vi "TTA_MATLAB_RX_Perform1RFIC1RxOutputPowerTest.vi"(0 "Channel":string(combo), 1 "MXG VISA Resource In":refnum<visa-resource-name>, 2 "EXA VISA Resource":refnum<visa-resource-name>, 5 "Rx":string(combo), 11 "error in":errorcluster) -> (4 "Output Power\nResults":T1, 12 "MXG VISA Resource Out":refnum<visa-resource-name>, 13 "EXA VISA Resource Out":refnum<visa-resource-name>, 15 "error out":errorcluster)   [LabVIEW 2016]
uses:
  TTA_Globals/TTA_Global_Complete_Settings.vi
panel:
  out "End Temp":dbl
  out "Start Temp":dbl
  out "In Range?":bool[](array[boolean])
  out "Amp Max\nSpec (dBm)":dbl
  out "Amp Min\nSpec (dBm)":dbl
  out "Frequency":dbl[](array[numeric])
  out "Amplitude":dbl[](array[numeric])
  out "IF Index":i32
  in  "PALLinearization Values":T2
  out "Rx#":i32
  out "CH#":i32
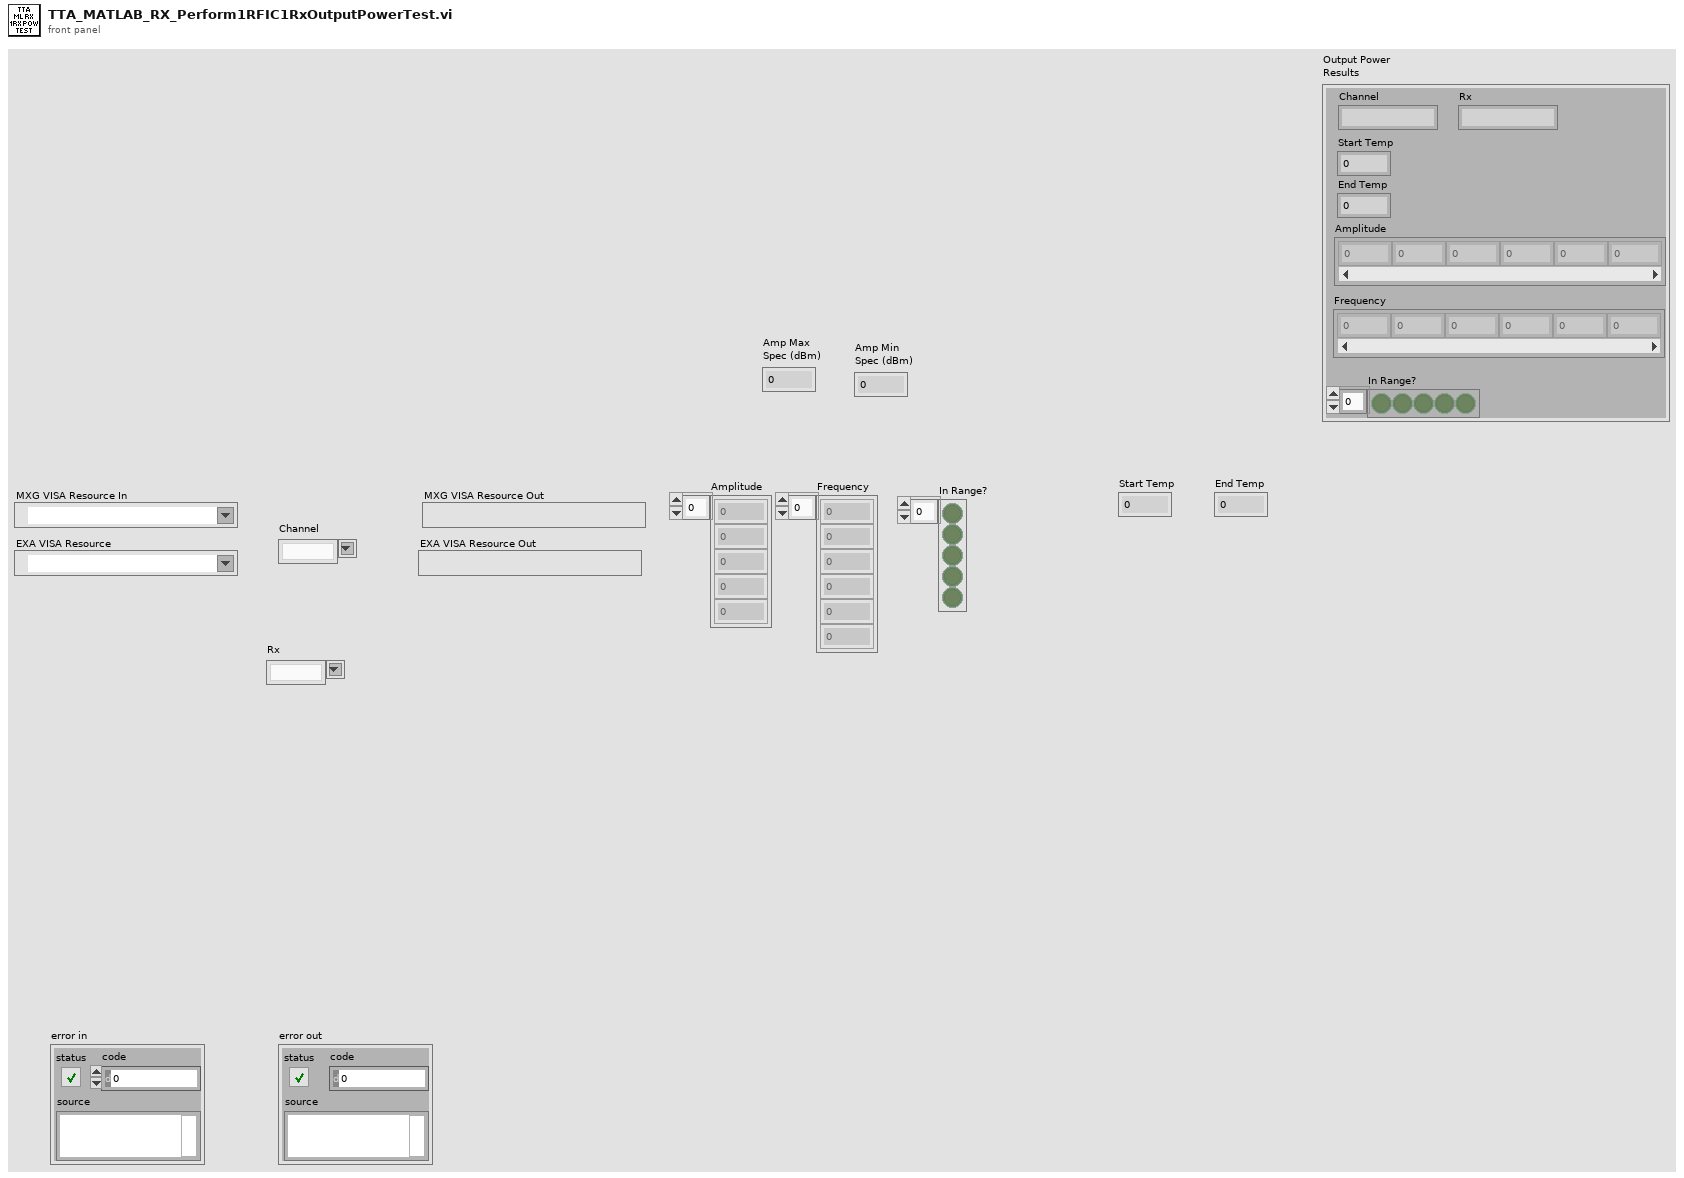
[diagram p1: front panel]
types:
  T1 = cluster{"Channel":string, "Rx":string, "Start Temp":dbl, "End Temp":dbl, "Amplitude":dbl[], "Frequency":dbl[], "In Range?":bool[]}
  T2 = cluster{"Tx IF Offsets":dbl[], "ACPR Filename":string, "Sampling Rate":dbl, "TxIF_Freq":dbl, "Power (dBm)":dbl, "IF Frequency Sweep (MHz)":dbl[], "BDSFreq":dbl, "Amplitude Range\nMax(dBm)":dbl, "Amplitude Range\nMin(dBm)":dbl, "CAL Amplitude\nIncrement(dB)":dbl, "CAL Amplitude\nDecrement (dB)":dbl, "Amplitude Least\nCriteria (dBm)":dbl}
  T3 = typedef "TTA_Control_Complete_Settings_Cluster.ctl" = cluster{"Brief Cluster":cluster{"STM Firmware File":string, "STM Firmware Address":string, "Required SW Version":string, "Template Used":string}, "Instrument Setting Cluster":cluster{"BDSFreq":dbl, "BDS Amp":dbl, "TxRFCal_Freq":dbl, "TxRFCal_Amp":dbl, "RxRFCal_Freq":dbl, "RxRFCal_Freq":dbl, "TxIF_Freq":dbl, "TxIF_Amp":dbl, "Tx_Output_Power_Signal_Freq":dbl, "Tx_ACPR_Signal_Freq":dbl, "Rx_RF_Freq":dbl, "Rx_RF_Amp":dbl, "Rx_Output_Power_Signal_Freq":dbl, "Rx_Output_Power_Sense_Freq":dbl}, "PAL Calibration\nInputs Cluster":cluster{"Amplitude Range\nMax(dBm)":dbl, "Amplitude Range\nMin(dBm)":dbl, "Amplitude Least\nCriteria (dBm)":dbl, "Frequency 1":dbl, "Frequency 2":dbl, "Frequency 3":dbl, "CAL Amplitude\nDecrement (dB)":dbl, "CAL Amplitude\nIncrement(dB)":dbl, "DownloadFile":string}, "TxOffset Cal Cluster":cluster{"Tx1 Offset (dB)":dbl, "Tx2 Offset (dB)":dbl, "Tx3 Offset (dB)":dbl, "Tx4 Offset (dB)":dbl, "Total RF Tx Loss (dB)":dbl}, "RxOffset Cal Cluster":cluster{"Rx1 Offset (dB)":dbl, "Rx2 Offset (dB)":dbl, "Rx3 Offset (dB)":dbl, "Rx4 Offset (dB)":dbl, "Total RF Rx Loss (dB)":dbl}, "TX Output Power Settings Cluster":cluster{"Frequency Sweep (MHz)":dbl[], "Sig Gen \nPower (dBm)":dbl, "Span (kHz)":dbl, "RBW (Hz)":dbl, "Ref Level (dBm)":dbl, "Low Power \nLimit":dbl, "High Power \nLimit":dbl, "DigAtt Max":dbl, "DigAtt Min":dbl}, "Tx ACPR Settings Cluster":cluster{"ACPR Filename":string, "Sampling Rate":dbl, "Power (dBm)":dbl, "IF Frequency Sweep (MHz)":dbl[], "State Name":string, "Mechanical\nAttenuation":dbl, "RefLevel Offset":dbl, "Amplitude Range\nMax (dBm)":dbl, "Amplitude Range\nMin (dBm)":dbl, "Cal Amp \nIncrement (dB)":dbl, "Cal Amp\nDecrement (dB)":dbl}, "Power Cal Cluster":cluster{"Power List (dBm)":dbl[], "Frequency (MHz)":dbl[], "Cal Decrement (dB)":dbl, "Cal Increment (dB)":dbl}, "Rx Received Power Settings Cluster":cluster{"Frequency Sweep (MHz)":dbl[], "Power (dBm)":dbl, "Span (kHz)":dbl, "RBW (Hz)":dbl, "Ref Level":dbl, "Low Power \nLimit (dBm)":dbl, "High Power\nLimit (dBm)":dbl}, "Tx Output Power Criteria Cluster":cluster{"CH1-TX1 \nMin":dbl, "CH1-TX1\nMax":dbl, "CH1-TXx3\nMin ":dbl, "CH1-TXx3\nMax":dbl, "CH2-TX1\nMin":dbl, "CH2-TX1\nMax":dbl, "CH2-TXx3\nMin":dbl, "CH2-TXx3\nMax":dbl}, "Tx ACPR Criteria Cluster":cluster{"Min Inband":dbl, "Max Close Outband":dbl, "Max Far Outband":dbl}, "Rx Output Power Criteria Cluster":cluster{"CH1-RX1 \nMin":dbl, "CH1-RX1 \nMax":dbl, "CH1-RXx3 \nMin":dbl, "CH1-RXx3\nMax":dbl, "CH2-RX1\nMin":dbl, "CH2-RX1\nMax":dbl, "CH2-RXx3\nMin":dbl, "CH2-RXx3\nMax":dbl}}
  T4 = cluster{"BDSFreq":dbl, "BDS Amp":dbl, "TxRFCal_Freq":dbl, "TxRFCal_Amp":dbl, "RxRFCal_Freq":dbl, "RxRFCal_Freq":dbl, "TxIF_Freq":dbl, "TxIF_Amp":dbl, "Tx_Output_Power_Signal_Freq":dbl, "Tx_ACPR_Signal_Freq":dbl, "Rx_RF_Freq":dbl, "Rx_RF_Amp":dbl, "Rx_Output_Power_Signal_Freq":dbl, "Rx_Output_Power_Sense_Freq":dbl}
  T5 = cluster{"Rx1 Offset (dB)":dbl, "Rx2 Offset (dB)":dbl, "Rx3 Offset (dB)":dbl, "Rx4 Offset (dB)":dbl, "Total RF Rx Loss (dB)":dbl}
  T6 = cluster{"Frequency Sweep (MHz)":dbl[], "Power (dBm)":dbl, "Span (kHz)":dbl, "RBW (Hz)":dbl, "Ref Level":dbl, "Low Power \nLimit (dBm)":dbl, "High Power\nLimit (dBm)":dbl}
  T7 = cluster{"CH1-RX1 \nMin":dbl, "CH1-RX1 \nMax":dbl, "CH1-RXx3 \nMin":dbl, "CH1-RXx3\nMax":dbl, "CH2-RX1\nMin":dbl, "CH2-RX1\nMax":dbl, "CH2-RXx3\nMin":dbl, "CH2-RXx3\nMax":dbl}
  T8 = enum16{"TX1", "TX2", "TX3", "TX4", "TXx3", "TXx4", "RX1", "RX2", "RX3", "RX4", "RXx3", "RXx4", "RFCal"}
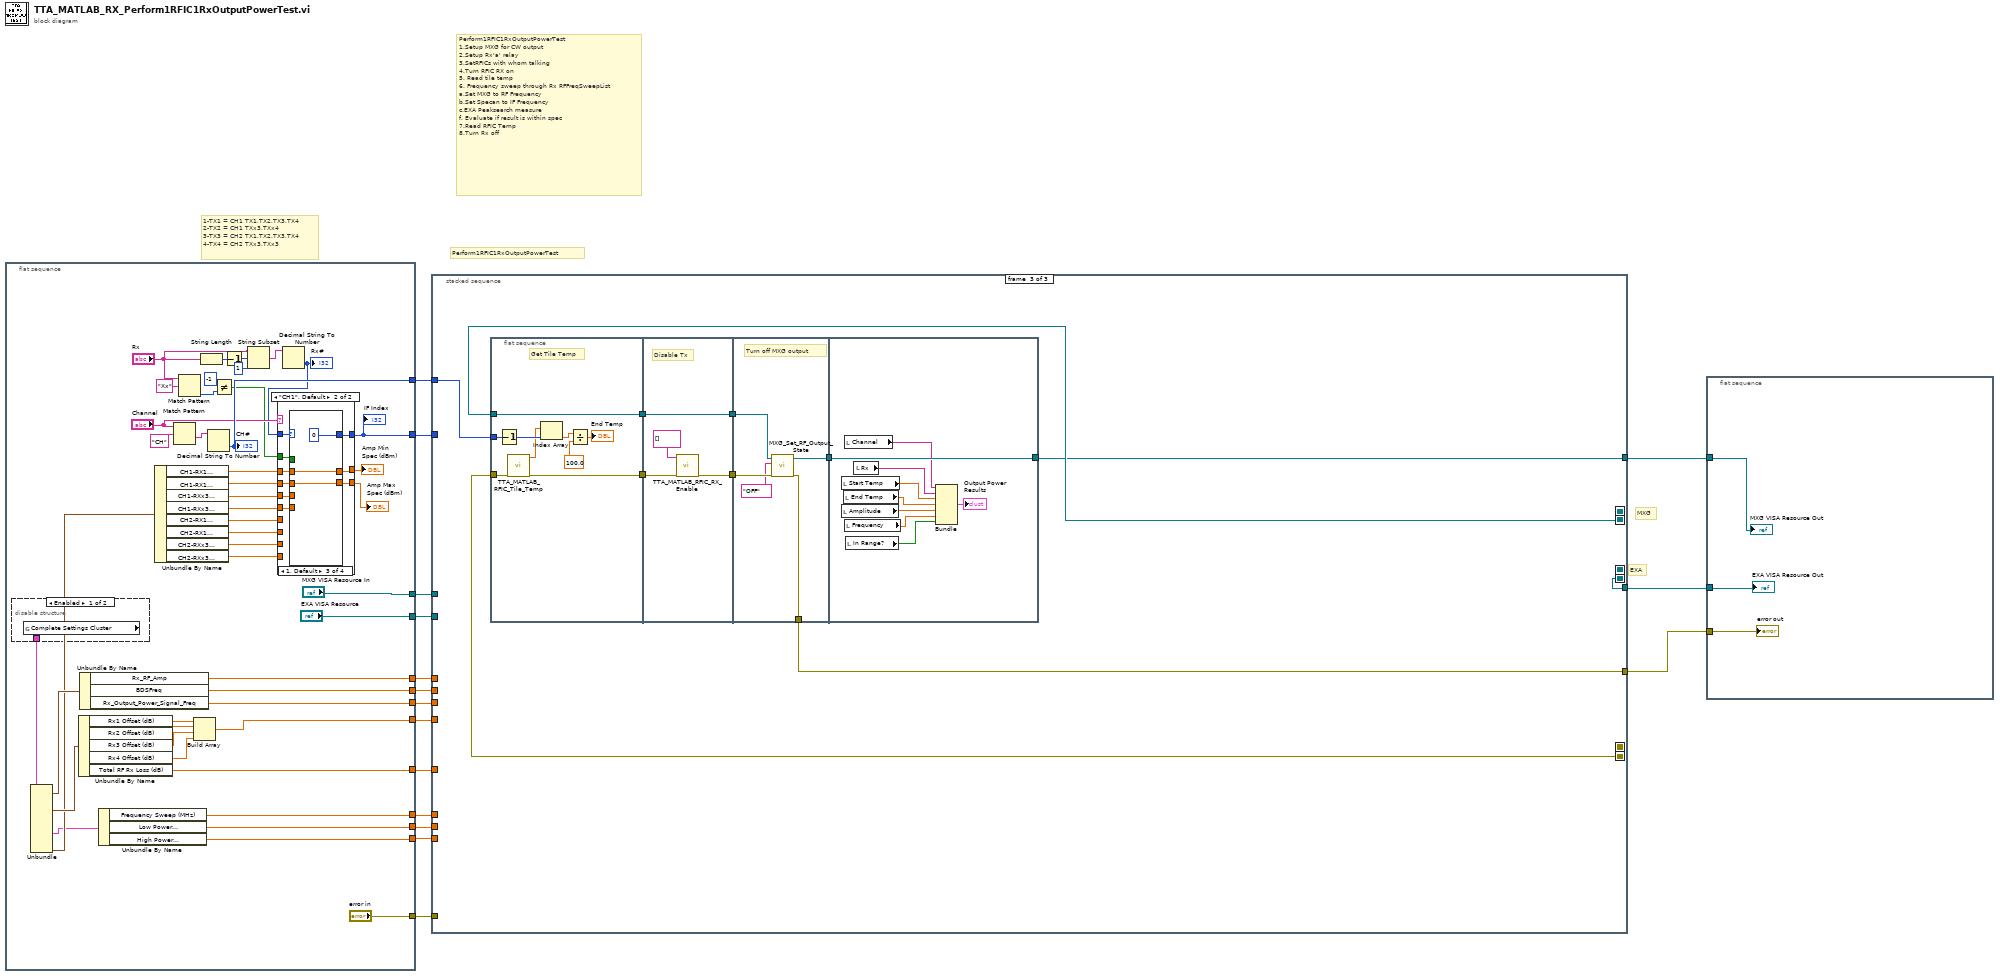
[diagram p0: block diagram]
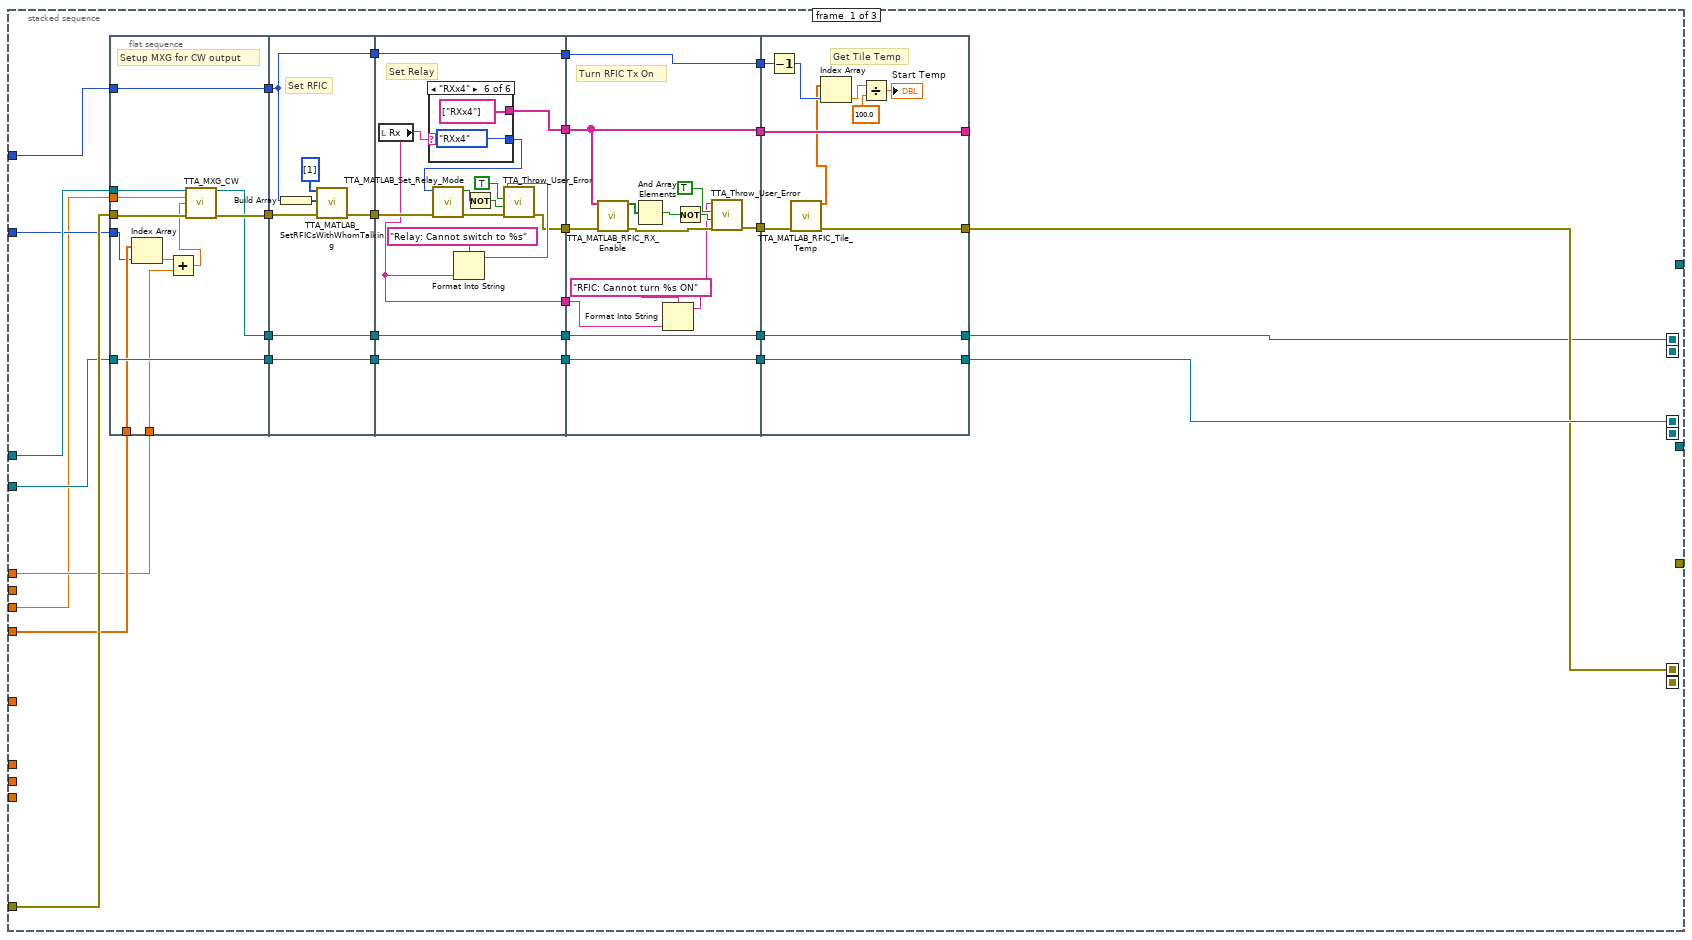
[diagram p2: hidden frame]
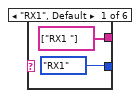
[diagram p3: hidden frame]
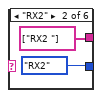
[diagram p4: hidden frame]
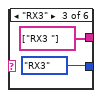
[diagram p5: hidden frame]
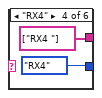
[diagram p6: hidden frame]
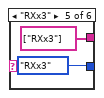
[diagram p7: hidden frame]
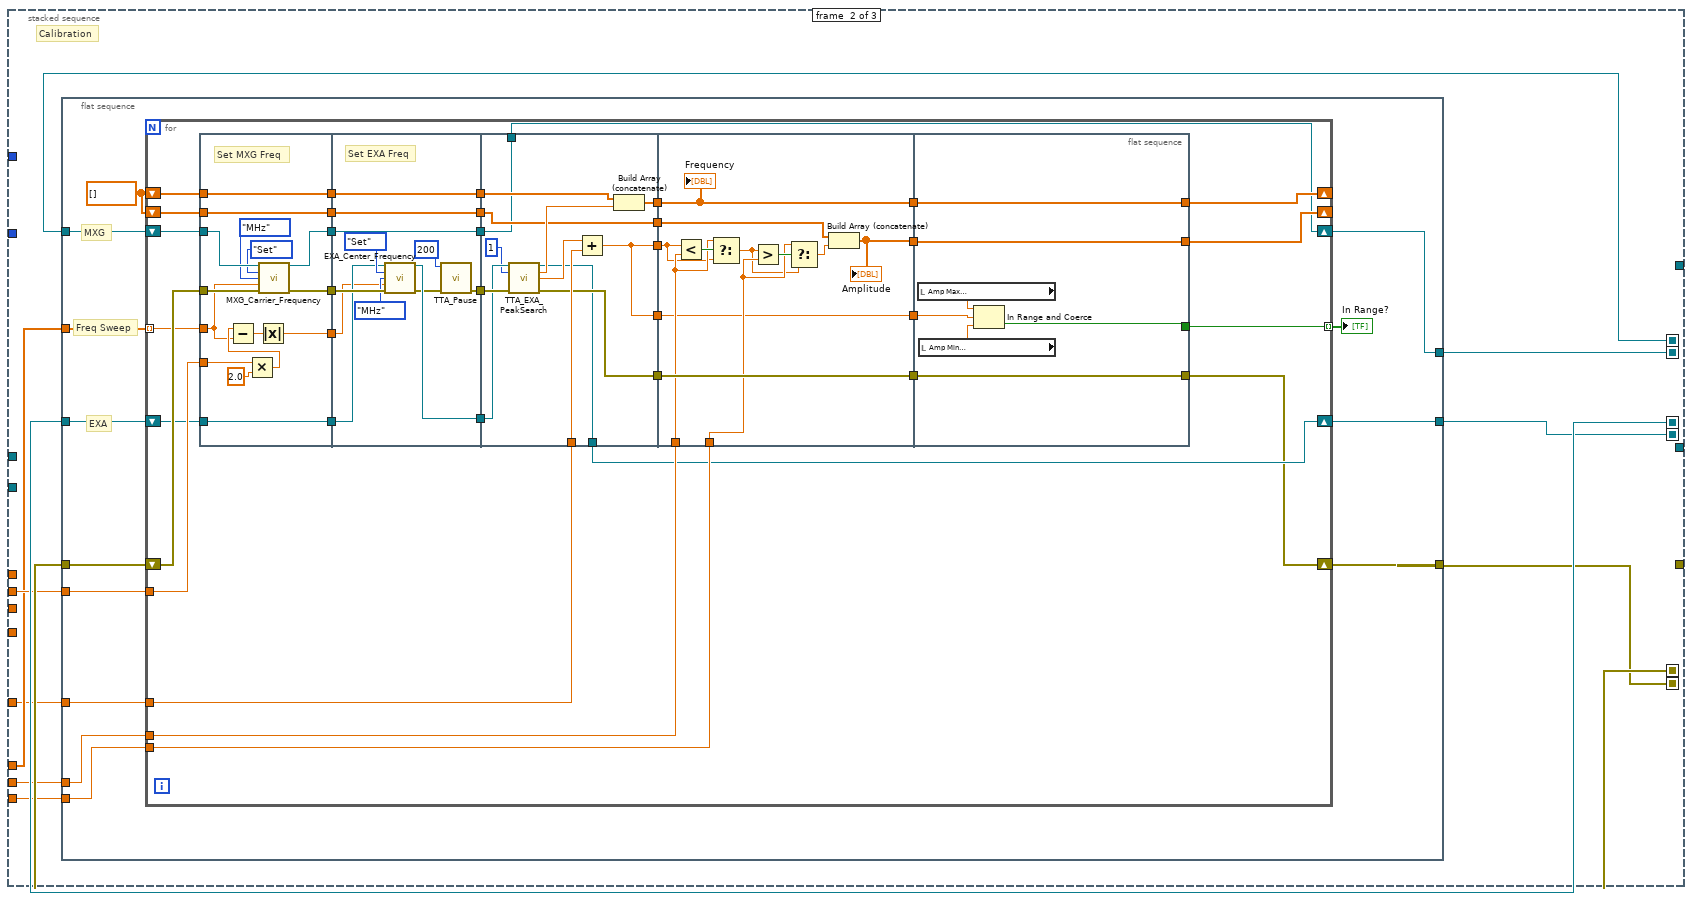
[diagram p8: hidden frame]
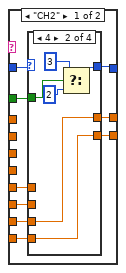
[diagram p9: hidden frame]
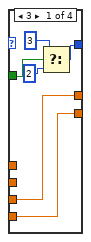
[diagram p10: hidden frame]
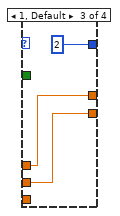
[diagram p11: hidden frame]
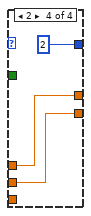
[diagram p12: hidden frame]
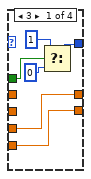
[diagram p13: hidden frame]
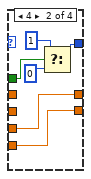
[diagram p14: hidden frame]
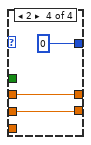
[diagram p15: hidden frame]
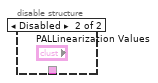
[diagram p16: hidden frame]
diagram:
  # "Perform1RFIC1RxOutputPowerTest\n1.Setup MXG for CW output\n2.Setup Rx'a' relay\n3.SetRFICs with whom talking\n4.Turn RFIC RX on\n5. Read tile temp\n6. Frequency sweep through Rx RFFreqSweepList\na.Set MXG to RF Frequency\nb.Set Specan to IF Frequency\nc.EXA Peaksearch measure\nf. Evaluate if result is within spec\n7.Read RFIC Temp\n8.Turn Rx off"
  # "Perform1RFIC1RxOutputPowerTest"
  # "1-TX1 = CH1 TX1,TX2,TX3,TX4\n2-TX2 = CH1 TXx3,TXx4\n3-TX3 = CH2 TX1,TX2,TX3,TX4\n4-TX4 = CH2 TXx3,TXx3"
  # "EXA"
  # "MXG"
  n1 = flat-sequence {
    tunnel: ["error in"] -> w16
    tunnel: ["MXG VISA Resource In"] -> w14
    tunnel: ["EXA VISA Resource"] -> w13
    tunnel: [w56] -> w15
    tunnel: [w43] -> w10
    tunnel: [w44] -> w9
    tunnel: [w49] -> w8
    tunnel: [w35] -> w7
    tunnel: [w34] -> w6
    tunnel: [w33] -> w5
    tunnel: [w32] -> w4
    tunnel: [w31] -> w3
    tunnel: [w30] -> w2
    frame #0 {
      n2 = disable-structure shown="Enabled" {
        disable-tunnel: [w116 _] -> w51
        frame Enabled {
          n3 = global read "TTA_Global_Complete_Settings.vi" "Complete Settings Cluster"() -> (w116:T3)
        }
        frame Disabled {
        }
      }
      n4 = Unbundle(w51) -> ("Instrument Setting Cluster"=w50:T4, "RxOffset Cal Cluster"=w19:T5, "Rx Received Power Settings Cluster"=w17:T6, "Rx Output Power Criteria Cluster"=w18:T7)  [unwired: 8 out]
      n5 = Unbundle By Name(w19) -> ("Rx1 Offset (dB)"=w48:dbl, "Rx2 Offset (dB)"=w47:dbl, "Rx3 Offset (dB)"=w46:dbl, "Rx4 Offset (dB)"=w45:dbl, "Total RF Rx Loss (dB)"=w32:dbl)
      n6 = Unbundle By Name(w50) -> ("Rx_RF_Amp"=w34:dbl, "BDSFreq"=w49:dbl, "Rx_Output_Power_Signal_Freq"=w43:dbl)
      n7 = Unbundle By Name(w17) -> ("Frequency Sweep (MHz)"=w33:dbl[], "Low Power \nLimit (dBm)"=w31:dbl, "High Power\nLimit (dBm)"=w30:dbl)
      n8 = Unbundle By Name(w18) -> ("CH1-RX1 \nMin"=w29:dbl, "CH1-RX1 \nMax"=w28:dbl, "CH1-RXx3 \nMin"=w27:dbl, "CH1-RXx3\nMax"=w26:dbl, "CH2-RX1\nMin"=w25:dbl, "CH2-RX1\nMax"=w24:dbl, "CH2-RXx3\nMin"=w23:dbl, "CH2-RXx3\nMax"=w22:dbl)
      n9 = Match Pattern(string="Channel", regular expression="CH") -> (after substring=w57:string)  [unwired: 1 in, 3 out]
      n10 = Match Pattern(string="Rx", regular expression="Xx") -> (offset past match=w38:i32)  [unwired: 1 in, 3 out]
      n11 = Build Array(w48, w47, w46, w45) -> (w44:dbl[])
      n12 = String Length(string="Rx") -> (length=w55:i32)
      n13 = Decimal String To Number(string=w57) -> (number=w56:i32)  [unwired: 2 in, 1 out]
      "CH#" <- w56
      n14 = Not Equal?(x=-1, y=w38) -> (x != y?=w36:bool)
      n15 = Decrement(x=w55) -> (x-1=w54:i32)
      n16 = String Subset(string="Rx", offset (0)=w54, length (rest)=1 ("length (rest)")) -> (substring=w52:string)
      n17 = Decimal String To Number(string=w52) -> (number=w41:i32)  [unwired: 2 in, 1 out]
      "Rx#" <- w41
      n18 = case shown="\"CH1\", Default" "Channel" {
        tunnel: w41 -> [w69 w97]
        tunnel: [w70 w96] -> w35
        tunnel: w36 -> [w68 w95]
        tunnel: w29 -> [_ w94]
        tunnel: w28 -> [_ w93]
        tunnel: w27 -> [_ w92]
        tunnel: w26 -> [_ w91]
        tunnel: w25 -> [w67 _]
        tunnel: w24 -> [w66 _]
        tunnel: w23 -> [w65 _]
        tunnel: w22 -> [w64 _]
        tunnel: [w63 w90] -> w21
        tunnel: [w62 w89] -> w20
        frame "CH2" {
          n19 = case shown="4" w69 {
            tunnel: [w74 w80 2 2] -> w70
            tunnel: w68 -> [w73 w79 _ _]
            tunnel: w67 -> [_ _ w84 w87]
            tunnel: [w72 w78 w84 w87] -> w63
            tunnel: w66 -> [_ _ w83 w86]
            tunnel: [w71 w77 w83 w86] -> w62
            tunnel: w65 -> [w72 w78 _ _]
            tunnel: w64 -> [w71 w77 _ _]
            frame 3 {
              n20 = Select(t=3, s=w73, f=2) -> (s? t:f=w74:i32)
            }
            frame 4 {
              n21 = Select(t=3, s=w79, f=2) -> (s? t:f=w80:i32)
            }
            frame 1, Default {
            }
            frame 2 {
            }
          }
        }
        frame "CH1", Default {
          n22 = case shown="1, Default" w97 {
            tunnel: [w101 w107 0 0] -> w96
            tunnel: w95 -> [w100 w106 _ _]
            tunnel: [w99 w105 w111 w114] -> w90
            tunnel: w94 -> [_ _ w111 w114]
            tunnel: [w98 w104 w110 w113] -> w89
            tunnel: w93 -> [_ _ w110 w113]
            tunnel: w92 -> [w99 w105 _ _]
            tunnel: w91 -> [w98 w104 _ _]
            frame 3 {
              n23 = Select(t=1, s=w100, f=0) -> (s? t:f=w101:i32)
            }
            frame 4 {
              n24 = Select(t=1, s=w106, f=0) -> (s? t:f=w107:i32)
            }
            frame 1, Default {
            }
            frame 2 {
            }
          }
        }
      }
      "IF Index" <- w35
      "Amp Min\nSpec (dBm)" <- w21
      "Amp Max\nSpec (dBm)" <- w20
    }
  }
  n25 = stacked-sequence {
    seq-local: [w121 _ _] -> [_ w227 _]
    seq-local: [w120 _ _] -> [_ w224 _]
    seq-local: [w134 _ _] -> [_ w226 _]
    seq-local: [_ w219 _] -> [_ _ w346]
    seq-local: [_ w217 _] -> [_ _ w343]
    seq-local: [_ w218 _] -> [_ _ w339]
    tunnel: w16 -> [w146 _ _]
    tunnel: w15 -> [w145 _ w336]
    tunnel: w14 -> [w143 _ _]
    tunnel: w13 -> [w142 _ _]
    tunnel: [_ _ w339] -> w12
    tunnel: [_ _ w338] -> w11
    tunnel: w10 -> [w126 _ _]
    tunnel: w9 -> [w128 _ _]
    tunnel: w8 -> [_ w225 _]
    tunnel: w7 -> [w129 _ _]
    tunnel: w6 -> [w127 _ _]
    tunnel: w5 -> [_ w223 _]
    tunnel: w4 -> [_ w222 _]
    tunnel: w3 -> [_ w221 _]
    tunnel: w2 -> [_ w220 _]
    tunnel: [_ _ w340] -> w1
    frame #0 {
      n26 = flat-sequence {
        tunnel: w142 -> [w157]
        tunnel: w143 -> [w154]
        tunnel: w145 -> [w158]
        tunnel: w146 -> [w156]
        tunnel: [w155] -> w133
        tunnel: [w158] -> w132
        tunnel: [w147] -> w131
        tunnel: [w157] -> w130
        tunnel: w129 -> [w152]
        tunnel: w128 -> [w153]
        tunnel: w127 -> [w151]
        tunnel: w126 -> [w148]
        tunnel: [w162] -> w144
        tunnel: [w161] -> w141
        tunnel: [w160] -> w140
        tunnel: w133 -> [w165]
        tunnel: w132 -> [w159]
        tunnel: w131 -> [w161]
        tunnel: w130 -> [w160]
        tunnel: [w159] -> w119
        tunnel: w144 -> [w179]
        tunnel: w141 -> [w171]
        tunnel: w140 -> [w169]
        tunnel: [w171] -> w139
        tunnel: [w167] -> w138
        tunnel: [w170] -> w137
        tunnel: [w169] -> w136
        tunnel: [w168] -> w135
        tunnel: w119 -> [w166]
        tunnel: [w166] -> w118
        tunnel: w139 -> [w194]
        tunnel: w138 -> [w198]
        tunnel: w137 -> [w197]
        tunnel: w136 -> [w196]
        tunnel: w135 -> [w195]
        tunnel: [w196] -> w125
        tunnel: [w198] -> w124
        tunnel: [w194] -> w123
        tunnel: [w193] -> w122
        tunnel: w118 -> [w192]
        tunnel: [w192] -> w117
        tunnel: [w214] -> w120
        tunnel: [w215] -> _
        tunnel: [w216] -> w134
        tunnel: w125 -> [w216]
        tunnel: w124 -> [w215]
        tunnel: w123 -> [w214]
        tunnel: w122 -> [w213]
        tunnel: [w212] -> w121
        tunnel: w117 -> [w210]
        frame #0 {
          # "Setup MXG for CW output"
          n27 = Index Array(array=w153, index=w152) -> (element=w150:dbl)
          n28 = Add(x=w150, y=w151) -> (x+y=w149:dbl)
          n29 = call "TTA_MXG_CW.vi"("VISA resource In"=w154, "Frequency (MHz)"=w148, "Output Power\nLevel (dBm)"=w149, "error in"=w156) -> ("VISA resource Out"=w147:refnum<visa-resource-name>, "error out"=w155:errorcluster)  [unwired: 10 in]
        }
        frame #1 {
          # "Set RFIC"
          n30 = Build Array(w159) -> (w163:i32[])
          n31 = call "TTA_MATLAB_SetRFICsWithWhomTalking.vi"("Panel Array"=i32[] [1], "RFIC Array"=w163, "error in"=w165) -> ("error out"=w162:errorcluster)  [unwired: 12 in]
        }
        frame #2 {
          # "Set Relay"
          n32 = local read "Rx"() -> (w168:string)
          n33 = case shown="\"RXx4\"" w168 {
            tunnel: [T8."RX1" ("Mode") T8."RX2" ("Mode") T8."RX3" ("Mode") T8."RX4" ("Mode") T8."RXx3" ("Mode") T8."RXx4" ("Mode")] -> w178
            tunnel: [string[] ["RX1 "] ("Channels") string[] ["RX2 "] ("Channels") string[] ["RX3 "] ("Channels") string[] ["RX4 "] ("Channels") string[] ["RXx3"] ("Channels") string[] ["RXx4"] ("Channels")] -> w167
            frame "RX1", Default {
            }
            frame "RX2" {
            }
            frame "RX3" {
            }
            frame "RX4" {
            }
            frame "RXx3" {
            }
            frame "RXx4" {
            }
          }
          n34 = call "TTA_MATLAB_Set_Relay_Mode.vi"("error in"=w179, "Mode"=w178) -> ("error out"=w177:errorcluster, "Success"=w176:bool)  [unwired: 8 in]
          n35 = Format Into String(format string="Relay: Cannot switch to %s", w168) -> (resulting string=w172:string)  [unwired: 2 in, 1 out]
          n36 = Not(x=w176) -> (.not. x?=w175:bool)
          n37 = call "TTA_Throw_User_Error.vi"("error in"=w177, "Error?"=w175, "Stop Execution on Fail"=TRUE, "Error Message"=w172) -> ("error out"=w170:errorcluster)  [unwired: 7 in]
        }
        frame #3 {
          # "Turn RFIC Tx On"
          n38 = call "TTA_MATLAB_RFIC_RX_Enable.vi"("Channels"=w198, "error in"=w197) -> ("SuccessComm"=w205:bool[], "error out"=w201:errorcluster)  [unwired: 12 in]
          n39 = And Array Elements(Boolean array=w205) -> (logical AND=w202:bool)
          n40 = Format Into String(format string="RFIC: Cannot turn %s ON", w195) -> (resulting string=w199:string)  [unwired: 2 in, 1 out]
          n41 = Not(x=w202) -> (.not. x?=w203:bool)
          n42 = call "TTA_Throw_User_Error.vi"("error in"=w201, "Error?"=w203, "Stop Execution on Fail"=TRUE, "Error Message"=w199) -> ("error out"=w193:errorcluster)  [unwired: 7 in]
        }
        frame #4 {
          # "Get Tile Temp"
          n43 = Decrement(x=w210) -> (x-1=w209:i32)
          n44 = call "TTA_MATLAB_RFIC_Tile_Temp.vi"("error in"=w213) -> ("Results"=w208:dbl[], "error out"=w212:errorcluster)  [unwired: 11 in, 2 out]
          n45 = Index Array(array=w208, index=w209) -> (element=w207:dbl)
          n46 = Divide(x=w207, y=100.0) -> (x/y=→"Start Temp":dbl)
        }
      }
    }
    frame #1 {
      # "Calibration"
      n47 = flat-sequence {
        tunnel: w227 -> [w240]
        tunnel: w226 -> [w239]
        tunnel: [w238] -> w218
        tunnel: [w237] -> w219
        tunnel: w225 -> [w236]
        tunnel: w223 -> [w235]
        tunnel: w224 -> [w234]
        tunnel: w222 -> [w233]
        tunnel: w221 -> [w231]
        tunnel: w220 -> [w230]
        tunnel: [w229] -> w217
        frame #0 {
          w232 = dbl[] []
          # "Freq Sweep"
          # "EXA"
          # "MXG"
          n48 = for {
            shift-right: [w247] -> w237
            shift-left: w240 -> [w274]
            shift-right: [w248] -> w238
            shift-left: w239 -> [w273]
            tunnel: w236 -> [w276]
            tunnel: w235 -> [w272] mode=indexing
            shift-right: [w249] -> w229
            shift-left: w234 -> [w275]
            tunnel: w233 -> [w264]
            shift-right: [w263] -> _
            shift-left: w232 -> [w258]
            shift-right: [w262] -> _
            shift-left: w232 -> [w261]
            tunnel: w231 -> [w253]
            tunnel: w230 -> [w252]
            tunnel: [w241] -> w228 mode=indexing
            n49 = flat-sequence {
              tunnel: w272 -> [w277]
              tunnel: w276 -> [w287]
              tunnel: w275 -> [w290]
              tunnel: w274 -> [w291]
              tunnel: w273 -> [w282]
              tunnel: [w284] -> w271
              tunnel: [w283] -> w270
              tunnel: [w282] -> w269
              tunnel: [w281] -> w268
              tunnel: w261 -> [w280]
              tunnel: [w280] -> w259
              tunnel: w258 -> [w279]
              tunnel: [w279] -> w256
              tunnel: w271 -> [w299]
              tunnel: w270 -> [w303]
              tunnel: w269 -> [w301]
              tunnel: w268 -> [w297]
              tunnel: [w298] -> w267
              tunnel: [w297] -> w266
              tunnel: [w294] -> w265
              tunnel: [w293] -> w260
              tunnel: w259 -> [w293]
              tunnel: [w292] -> w257
              tunnel: w256 -> [w292]
              tunnel: w267 -> [w315]
              tunnel: w266 -> [w306]
              tunnel: w265 -> [w316]
              tunnel: w264 -> [w313]
              tunnel: w260 -> [w309]
              tunnel: w257 -> [w308]
              tunnel: [w311] -> w255
              tunnel: [w304] -> w254
              tunnel: [w308] -> w251
              tunnel: [w307] -> w250
              tunnel: [w306] -> w249
              tunnel: [w305] -> w248
              tunnel: [w304] -> w242
              tunnel: w255 -> [w328]
              tunnel: w254 -> [w325]
              tunnel: w253 -> [w326]
              tunnel: w252 -> [w323]
              tunnel: w251 -> [w320]
              tunnel: w250 -> [w318]
              tunnel: [w328] -> w246
              tunnel: [w318] -> w245
              tunnel: [w319] -> w244
              tunnel: [w317] -> w243
              tunnel: w242 -> [w317]
              tunnel: [w333] -> w263
              tunnel: [w334] -> w262
              tunnel: [w335] -> w247
              tunnel: w246 -> [w335]
              tunnel: w245 -> [w334]
              tunnel: w244 -> [w333]
              tunnel: w243 -> [w330]
              tunnel: [w329] -> w241
              frame #0 {
                # "Set MXG Freq"
                n50 = Multiply(x=w287, y=2.0) -> (x*y=w278:dbl)
                n51 = Subtract(x=w278, y=w277) -> (x-y=w285:dbl)
                n52 = Absolute Value(x=w285) -> (abs(x)=w284:dbl)
                n53 = call "MXG_Carrier_Frequency.vi"("VISA resource name"=w290, "Mode"=enum16{"Set", "Get"}."Set", "Units"=enum16{"Hz", "kHz", "MHz", "GHz"}."MHz", "Frequency"=w277, "error in"=w291) -> ("VISA resource name"=w281:refnum<visa-resource-name>, "error out"=w283:errorcluster)  [unwired: 8 in, 1 out]
              }
              frame #1 {
                # "Set EXA Freq"
                n54 = call "EXA_Center_Frequency.vi"("VISA resource name"=w301, "Mode"=enum16{"Set", "Get"}."Set", "Units"=enum16{"Hz", "kHz", "MHz", "GHz"}."MHz", "Frequency"=w299, "error in"=w303) -> ("VISA resource name"=w298:refnum<visa-resource-name>, "error out"=w296:errorcluster)  [unwired: 8 in, 1 out]
                n55 = call "TTA_Pause.vi"("error in"=w296, "Pause (ms)"=u32 200) -> ("error out"=w294:errorcluster)  [unwired: 9 in]
              }
              frame #2 {
                n56 = call "TTA_EXA_PeakSearch.vi"("VISA resource In"=w315, "Marker\nNumber"=1 ("Marker\nNumber"), "error in"=w316) -> ("VISA resource Out"=w305:refnum<visa-resource-name>, "Frequency (Hz)"=w310:dbl, "Amplitude (dBm)"=w312:dbl, "error out"=w311:errorcluster)  [unwired: 9 in]
                n57 = Add(x=w312, y=w313) -> (x+y=w304:dbl)
                n58 = Build Array (concatenate)(w309, w310) -> (w307:dbl[])
              }
              frame #3 {
                n59 = Less?(x=w325, y=w326) -> (x < y?=w327:bool)
                n60 = Select(t=w326, s=w327, f=w325) -> (s? t:f=w322:dbl)
                n61 = Greater?(x=w322, y=w323) -> (0:w324:bool)
                n62 = Select(t=w323, s=w324, f=w322) -> (s? t:f=w321:dbl)
                n63 = Build Array (concatenate)(w320, w321) -> (w319:dbl[])
                "Amplitude" <- w319
                "Frequency" <- w318
              }
              frame #4 {
                n64 = local read "Amp Max\nSpec (dBm)"() -> (w332:dbl)
                n65 = local read "Amp Min\nSpec (dBm)"() -> (w331:dbl)
                n66 = In Range and Coerce(upper limit=w332, x=w330, lower limit=w331) -> (In Range?=w329:bool)  [unwired: 1 out]
              }
            }
          }
          "In Range?" <- w228
        }
      }
    }
    frame #2 {
      n67 = flat-sequence {
        tunnel: w346 -> [w353]
        tunnel: [w355] -> w345
        tunnel: w343 -> [w352]
        tunnel: [w352] -> w341
        tunnel: w336 -> [w350]
        tunnel: w345 -> [w358]
        tunnel: [w357] -> w344
        tunnel: [w356] -> w342
        tunnel: w341 -> [w356]
        tunnel: w344 -> [w364]
        tunnel: w342 -> [w363]
        tunnel: [w360] -> w338
        tunnel: [w361] -> w337
        tunnel: [w373] -> w340
        tunnel: w337 -> [w373]
        frame #0 {
          # "Get Tile Temp"
          n68 = Decrement(x=w350) -> (x-1=w351:i32)
          n69 = call "TTA_MATLAB_RFIC_Tile_Temp.vi"("error in"=w353) -> ("Results"=w349:dbl[], "error out"=w355:errorcluster)  [unwired: 11 in, 2 out]
          n70 = Index Array(array=w349, index=w351) -> (element=w348:dbl)
          n71 = Divide(x=w348, y=100.0) -> (x/y=→"End Temp":dbl)
        }
        frame #1 {
          # "Disable Tx"
          n72 = call "TTA_MATLAB_RFIC_RX_Enable.vi"("Channels"=string[] [], "error in"=w358) -> ("error out"=w357:errorcluster)  [unwired: 12 in, 1 out]
        }
        frame #2 {
          # "Turn off MXG output"
          n73 = call "MXG_Set_RF_Output_State.vi"("error in"=w364, "RF Output State"="OFF", "VISA resource name"=w363) -> ("error out"=w360:errorcluster, "VISA resource name"=w361:refnum<visa-resource-name>)  [unwired: 7 in]
        }
        frame #3 {
          n74 = local read "Start Temp"() -> (w372:dbl)
          n75 = local read "Amplitude"() -> (w370:dbl[])
          n76 = local read "End Temp"() -> (w371:dbl)
          n77 = local read "Channel"() -> (w367:string)
          n78 = local read "Frequency"() -> (w369:dbl[])
          n79 = local read "In Range?"() -> (w368:bool[])
          n80 = local read "Rx"() -> (w366:string)
          n81 = Bundle("Channel"=w367, "Rx"=w366, "Start Temp"=w372, "End Temp"=w371, "Amplitude"=w370, "Frequency"=w369, "In Range?"=w368) -> (→"Output Power\nResults":T1)  [unwired: 1 in]
        }
      }
    }
  }
  n82 = flat-sequence {
    tunnel: w12 -> [w376]
    tunnel: w11 -> [w375]
    tunnel: w1 -> [w374]
    frame #0 {
      "error out" <- w375
      "MXG VISA Resource Out" <- w374
      "EXA VISA Resource Out" <- w376
    }
  }
